vi "ge_EditDBL.vi"(4 "CellSize":T2, 6 "ActiveCellPos":T1, 7 "String Value":string, 8 "error in":errorcluster, 11 "FP Ctrl":T3) -> (0 "error out":errorcluster, 1 "Discard?":bool)   [LabVIEW 2018]
uses:
  Custom Ctrls/ge_FPCtrlRefLabel.ctl
  <vilib>/Utility/miscctls.llb/LVBoundsTypeDef.ctl
  <vilib>/Utility/miscctls.llb/LVPositionTypeDef.ctl
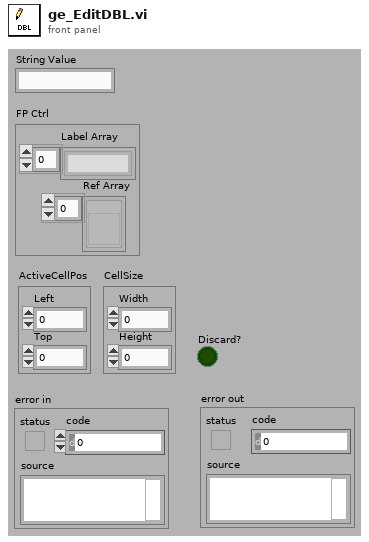
[diagram p1: front panel]
types:
  T1 = typedef "LVPositionTypeDef.ctl" = cluster{"Left":i32, "Top":i32}
  T2 = typedef "LVBoundsTypeDef.ctl" = cluster{"Width":u32, "Height":u32}
  T3 = typedef "ge_FPCtrlRefLabel.ctl" = cluster{"Label Array":string[], "Ref Array":refnum<vi>[]}
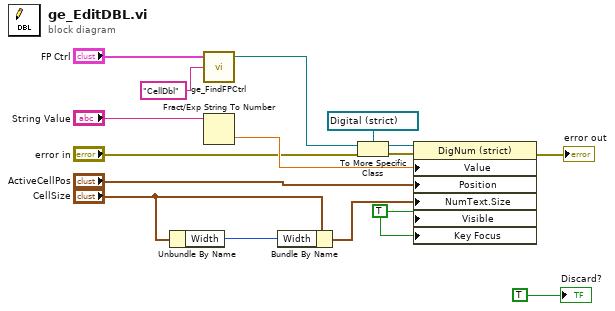
[diagram p0: block diagram]
diagram:
  w10 = TRUE ("Visible")
  n1 = Unbundle By Name("CellSize") -> ("Width"=w2:u32)
  n2 = call "ge_FindFPCtrl.vi"("Ctrl Name"="CellDbl" ("Name"), "FP Ctrl"="FP Ctrl") -> ("Ctrl Ref"=w4:refnum<vi>)  [unwired: 3 in]
  n3 = Fract/Exp String To Number(string="String Value") -> (number=w11:dbl)  [unwired: 3 in, 1 out]
  n4 = Bundle By Name(cluster="CellSize", "Width"=w2) -> (w12:T2)
  n5 = To More Specific Class(target class=refnum<vi> refnum ("reference"), reference=w4, error in="error in") -> (specific class reference=w7:refnum<vi>, error out=w8:errorcluster)
  n6 = property on="Property Node" class="DigNum (strict)"(reference=w7, error in=w8, "Value"=w11, "Position"="ActiveCellPos", "NumText.Size"=w12, "Visible"=w10, "Key Focus"=w10) -> (error out=→"error out":errorcluster)  [unwired: 1 out]
  "Discard?" <- TRUE ("Discard?")
